vi "Async Initialize.vi"(8 "error in (no error)":errorcluster, 10 "RT Configuration":T1={"Name"="", "Priority"=0, "CAN Session"="", "Frame Count"=0, "Frames"=[], "FPGA Session"=0, "XNET Settings"={"Database"="", "Cluster"="", "Port"="", "Baud rate [Bd]"=0, "Termination"=0, "CAN I/O Mode"=0, "FD Baud rate [Bd]"=500000, "Priority"=100, "Use Legacy"=FALSE, "FD ISO Mode"=0}, "Incoming Frame Session"="", "Incoming Session Invalid"=FALSE, "Incoming Signal Info"={"Signal_Valid_Values"=[], "Signal Names"=[], "Signal Settings Out"=[], "Frame Receive Time Values"=[], "ProtCtr Sig Values"=[]}, "Signal Values"=[]} {"Incoming Signal Info"."Signal Settings Out"."Protection Configuration"."CRC Channels"."Data Type" items=["Signed", "Unsigned", "IEEE Float"]; "XNET Settings"."FD ISO Mode" items=["ISO", "Non ISO", "ISO Legacy"]; "XNET Settings"."CAN I/O Mode" items=["CAN 2.0", "CAN FD", "CAN FD+BRS"]; "XNET Settings"."Termination" items=["Off", "On"]; "Frames"."Protection Configurations"."CRC Channels"."Data Type" items=["Signed", "Unsigned", "IEEE Float"]}, 11 "Process in":refnum<class "Process.lvclass">) -> (0 "error out":errorcluster, 2 "Execute":bool, 3 "Variables":T12={"Process Ref"=refnum, "Comm Ref"=refnum, "Data Refs"={"ProtectionsAndCounters.Ref"=refnum, "Signals.Ref"=refnum, "Status.Ref"=refnum, "Overrides"=refnum, "IncomingSignals.Ref"=refnum, "CtrandProtctnVld.Ref"=refnum, "RcvTime.Ref"=refnum, "TimeDiff.Ref"=refnum, "IncomingProtCtr.Ref"=refnum}, "Settings"={"Name"="", "Priority"=0, "CAN Session"="", "Frame Count"=0, "Frames"=[], "FPGA Session"=0, "XNET Settings"={"Database"="", "Cluster"="", "Port"="", "Baud rate [Bd]"=0, "Termination"=0, "CAN I/O Mode"=0, "FD Baud rate [Bd]"=500000, "Priority"=100, "Use Legacy"=FALSE, "FD ISO Mode"=0}, "Incoming Frame Session"="", "Incoming Session Invalid"=FALSE, "Incoming Signal Info"={"Signal_Valid_Values"=[], "Signal Names"=[], "Signal Settings Out"=[], "Frame Receive Time Values"=[], "ProtCtr Sig Values"=[]}, "Signal Values"=[]}, "Stream Refs"={"Addon"="", "Port"="", "Filter Ref"=refnum, "Default Filter"={"ID Filters"=[], "Direction Filter"=enum."Tx/Rx", "Type Filter"=enum."All"}, "Port Settings"={"Mode"=0, "Baud Rate"=0, "Termination"=0, "FD ISO Mode"=0, "FD Baud Rate"=0}}, "Signal Values"=[], "Incoming Signal Info"={"Signal_Valid_Values"=[], "Signal Names"=[], "Signal Settings Out"=[], "Frame Receive Time Values"=[], "ProtCtr Sig Values"=[]}, "Incoming Frame Session"="", "Incoming Session Invalid"=FALSE} {"Incoming Signal Info"."Signal Settings Out"."Protection Configuration"."CRC Channels"."Data Type" items=["Signed", "Unsigned", "IEEE Float"]; "Stream Refs"."Port Settings"."FD ISO Mode" items=["ISO", "Non ISO", "ISO Legacy"]; "Stream Refs"."Port Settings"."Termination" items=["Off", "On"]; "Stream Refs"."Port Settings"."Mode" items=["CAN 2.0", "CAN FD", "CAN FD+BRS"]; "Settings"."XNET Settings"."FD ISO Mode" items=["ISO", "Non ISO", "ISO Legacy"]; "Settings"."XNET Settings"."CAN I/O Mode" items=["CAN 2.0", "CAN FD", "CAN FD+BRS"]; "Settings"."XNET Settings"."Termination" items=["Off", "On"]})   [LabVIEW 2019, in "Protection and Counter Addon Engine.lvlib"]
uses:
  Protection and Counter Addon Engine.lvlib
  Types/RT Async Engine Variables.ctl
  <vilib>/NI/NIVS Inline Async API/_VS Inline Async API/Process/Process.lvclass
  <vilib>/NI/NI VeriStand Addon Network Comm/Engine/VeriStand Comm.lvclass
  Types/RT Data References.ctl
  <vilib>/NI/NIVS Inline Async API/_Data Access Engine/Data Access Engine/Types/Write.DVR.ctl
  <vilib>/NI/NIVS Inline Async API/_Data Access Engine/Access Type Classes/Write/Write.lvclass
  <vilib>/NI/NIVS Inline Async API/_Data Access Engine/Data Access Engine/Types/Read.DVR.ctl
  <vilib>/NI/NIVS Inline Async API/_Data Access Engine/Access Type Classes/Read/Read.lvclass
  Types/RT Async Engine Settings.ctl
  SubModules/Frame-Protection-Support/Source/Engine/Types/RT Frame Settings.ctl
  SubModules/Frame-Protection-Support/Source/Shared/Types/Exported Frame Type.ctl
  SubModules/Frame-Protection-Support/Source/Engine/Types/RT Protection Configuration.ctl
  SubModules/Frame-Protection-Support/Source/Shared/Types/Protection Type.ctl
  SubModules/Frame-Protection-Support/Source/Shared/Types/XNET Signal Configuration.ctl
  SubModules/Frame-Protection-Support/Source/Shared/Types/Exported Counter Settings.ctl
  SubModules/Frame-Protection-Support/Source/Shared/Types/Exported Event Trigger Type.ctl
  Addon Shared/Types/XNET Settings.ctl
  SubModules/Frame-Protection-Support/Source/Shared/Types/RT_Incoming_Signal_Info.ctl
  SubModules/Frame-Protection-Support/Source/Shared/Types/RT Exported Signal Settings.ctl
  SubModules/CAN-Streaming-Support/Source/Addon/Addon Engine/Types/Engine Stream Refs.ctl
  SubModules/CAN-Streaming-Support/Source/Addon/Addon Shared/Types/Direction Filter.ctl
  SubModules/CAN-Streaming-Support/Source/Addon/Addon Shared/Types/Type Filter.ctl
  SubModules/CAN-Streaming-Support/Source/Addon/Addon Shared/Types/Filter Parameters.ctl
  SubModules/CAN-Streaming-Support/Source/Addon/Addon Engine/Types/Engine Stream Port Settings.ctl
  <vilib>/NI/NI VeriStand Addon Network Comm/Engine/VeriStand Comm.lvclass/VeriStand Comm.ctl
  <vilib>/NI/NIVS Inline Async API/_VS Inline Async API/Process/Process.lvclass/Process.ctl
  <vilib>/NI/NIVS Inline Async API/_VS Inline Async API/Process/Data Member Access/Read Data Access.vi
  <vilib>/NI/NIVS Inline Async API/_VS Inline Async API/Error Handling Process/SubVIs/Error.ConvertArray.vi
  Addon Shared/SubVIs/GUID Lookup.vi
  <vilib>/Utility/SystemLogging/Write to System Log.vi
  <vilib>/NI/AMC/Create Message Queue.vi
  <vilib>/NI/STM/Connection Manager/TCP/Advanced/TCP Initialize Connection Manager (By Reference).vi
  <vilib>/NI/NIVS Inline Async API/_Data Access Engine/Data Access Engine/Methods/Read.Lookup.vi
  <vilib>/NI/NIVS Inline Async API/_Data Access Engine/Data Access Engine/Methods/Write.Lookup.vi
  <vilib>/NI/NIVS Inline Async API/_Data Access Engine/Data Access Engine/Data Access Engine.lvclass
  Addon Shared/Protection and Counter Addon Shared.lvlib
  SubModules/Frame-Protection-Support/Source/Shared/Protection and Counter Support Shared.lvlib
  SubModules/Frame-Protection-Support/Source/Engine/Protection and Counter Support Engine.lvlib
  SubModules/CAN-Streaming-Support/Source/Addon/Addon Shared/CAN Stream Support Shared.lvlib
  SubModules/CAN-Streaming-Support/Source/Addon/Addon Engine/CAN Stream Support Engine.lvlib
  <resource>/objmgr/xnet.rc
  <vilib>/NI VeriStand/Custom Device Tools/Custom Device Utility Library/Custom Device Utility Library.lvlib
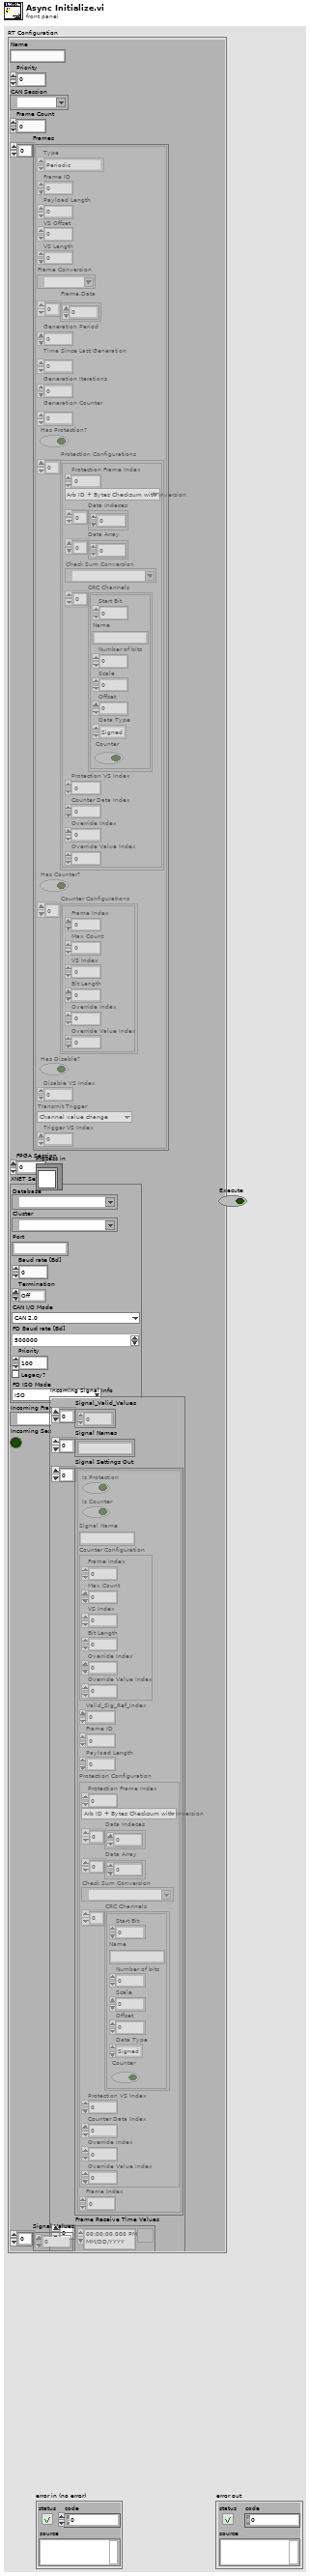
[diagram p1: front panel]
types:
  T1 = typedef "Protection and Counter Addon Engine.lvlib/RT Async Engine Settings.ctl" = cluster{"Name":string, "Priority":i32, "CAN Session":refnum<k21>, "Frame Count":i32, "Frames":T2[], "FPGA Session":u32, "XNET Settings":T9, "Incoming Frame Session":refnum<k21>, "Incoming Session Invalid":bool, "Incoming Signal Info":T10, "Signal Values":dbl[]}
  T2 = typedef "Protection and Counter Support Engine.lvlib/RT Frame Settings.ctl" = cluster{"Type":T3, "Frame ID":u32, "Payload Length":u32, "VS Offset":i32, "VS Length":i32, "Frame Conversion":refnum<k21>, "Frame.Data":dbl[], "Generation Period":u32, "Time Since Last Generation":u32, "Generation Iterations":u32, "Generation Counter":u32, "Has Protection?":bool, "Protection Configurations":T4[], "Has Counter?":bool, "Counter Configurations":T7[], "Has Disable?":bool, "Disable VS Index":i32, "Transmit Trigger":T8, "Trigger VS Index":i32}
  T3 = typedef "Protection and Counter Support Shared.lvlib/Exported Frame Type.ctl" = enum16{"Periodic", "Event", "Periodic/Event"}
  T4 = typedef "Protection and Counter Support Engine.lvlib/RT Protection Configuration.ctl" = cluster{"Protection Frame Index":i32, "Protection Type":T5, "Data Indeces":i32[], "Data Array":dbl[], "Check Sum Conversion":refnum<k21>, "CRC Channels":T6[], "Protection VS Index":i32, "Counter Data Index":i32, "Override Index":i32, "Override Value Index":i32}
  T5 = typedef "Protection and Counter Support Shared.lvlib/Protection Type.ctl" = enum16{"Arb ID + Bytes Checksum with Inversion", "Arb ID + Bytes CRC with Inversion", "Reversed Raw Signal Checksum with Inversion", "Concatenated Two's Compliment"}
  T6 = typedef "Protection and Counter Support Shared.lvlib/XNET Signal Configuration.ctl" = cluster{"Start Bit":i32, "Name":string, "Number of bits":i32, "Scale":dbl, "Offset":dbl, "Data Type":u32, "Counter":bool}
  T7 = typedef "Protection and Counter Support Shared.lvlib/Exported Counter Settings.ctl" = cluster{"Frame Index":i32, "Max Count":dbl, "VS Index":i32, "Bit Length":i64, "Override Index":i32, "Override Value Index":i32}
  T8 = typedef "Protection and Counter Support Shared.lvlib/Exported Event Trigger Type.ctl" = enum16{"Channel value change", "Trigger channel (not zero)", "Channel value change or trigger channel (not zero)", "Trigger channel (any value change)", "Channel value change or trigger channel (any value change)"}
  T9 = typedef "Protection and Counter Addon Shared.lvlib/XNET Settings.ctl" = cluster{"Database":refnum<k21>, "Cluster":refnum<k21>, "Port":string, "Baud rate [Bd]":u64, "Termination":u32, "CAN I/O Mode":u32, "FD Baud rate [Bd]":u64, "Priority":i32, "Use Legacy":bool, "FD ISO Mode":u32}
  T10 = typedef "RT_Incoming_Signal_Info.ctl" = cluster{"Signal_Valid_Values":dbl[], "Signal Names":string[], "Signal Settings Out":T11[], "Frame Receive Time Values":timestamp[], "ProtCtr Sig Values":dbl[]}
  T11 = typedef "RT Exported Signal Settings.ctl" = cluster{"Is Protection":bool, "Is Counter":bool, "Signal Name":string, "Counter Configuration":T7, "Valid_Sig_Ref_Index":i32, "Frame ID":u32, "Payload Length":u32, "Protection Configuration":T4, "Frame Index":i32}
  T12 = typedef "Protection and Counter Addon Engine.lvlib/RT Async Engine Variables.ctl" = cluster{"Process Ref":refnum<class "Process.lvclass">, "Comm Ref":refnum<class "VeriStand Comm.lvclass">, "Data Refs":T13, "Settings":T1, "Stream Refs":T16, "Signal Values":dbl[], "Incoming Signal Info":T10, "Incoming Frame Session":refnum<k21>, "Incoming Session Invalid":bool}
  T13 = typedef "Protection and Counter Addon Engine.lvlib/RT Data References.ctl" = cluster{"ProtectionsAndCounters.Ref":T14, "Signals.Ref":T15, "Status.Ref":T14, "Overrides":T15, "IncomingSignals.Ref":T14, "CtrandProtctnVld.Ref":T14, "RcvTime.Ref":T14, "TimeDiff.Ref":T14, "IncomingProtCtr.Ref":T14}
  T14 = typedef "Data Access Engine.lvlib/Data Access Engine.lvclass/Write.DVR.ctl" = refnum<data-value>
  T15 = typedef "Data Access Engine.lvlib/Data Access Engine.lvclass/Read.DVR.ctl" = refnum<data-value>
  T16 = typedef "CAN Stream Support Engine.lvlib/Engine Stream Refs.ctl" = cluster{"Addon":string, "Port":refnum<k21>, "Filter Ref":refnum<data-value>, "Default Filter":T17, "Port Settings":T20}
  T17 = typedef "CAN Stream Support Shared.lvlib/Filter Parameters.ctl" = cluster{"ID Filters":u32[], "Direction Filter":T18, "Type Filter":T19}
  T18 = typedef "CAN Stream Support Shared.lvlib/Direction Filter.ctl" = enum16{"Tx/Rx", "Rx", "Tx"}
  T19 = typedef "CAN Stream Support Shared.lvlib/Type Filter.ctl" = enum16{"All", "CAN Data", "CAN Remote", "CAN Bus Error", "CAN 2.0 Data", "CAN FD Data", "CAN FD+BRS Data", "J1939 Data", "Delay", "Log Trigger", "Start Trigger"}
  T20 = typedef "CAN Stream Support Engine.lvlib/Engine Stream Port Settings.ctl" = cluster{"Mode":u32, "Baud Rate":u64, "Termination":u32, "FD ISO Mode":u32, "FD Baud Rate":u64}
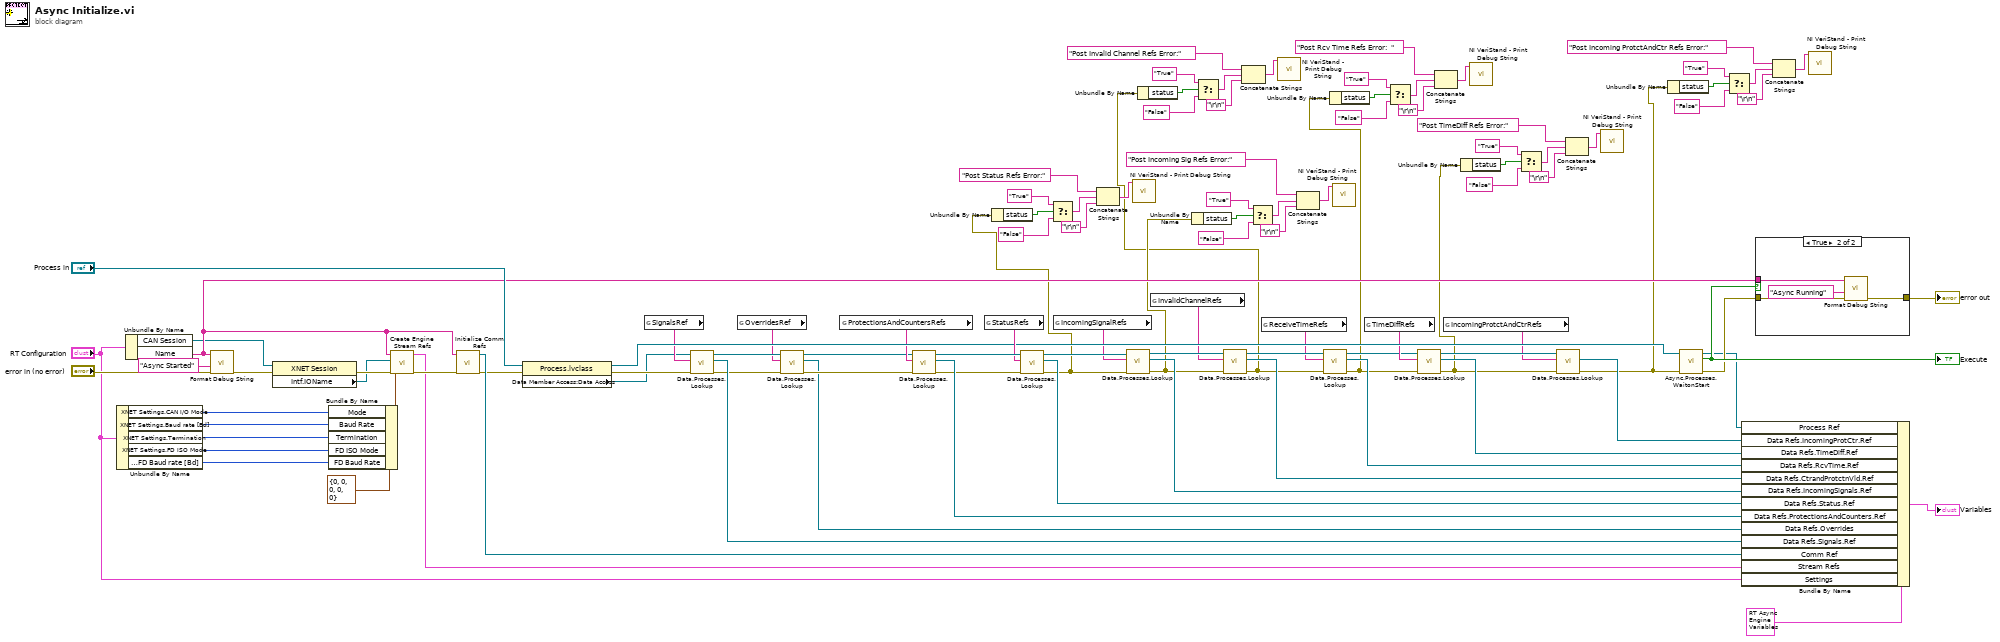
[diagram p0: block diagram]
diagram:
  n1 = Unbundle By Name("RT Configuration") -> ("XNET Settings.CAN I/O Mode"=w69:u32, "XNET Settings.Baud rate [Bd]"=w66:u64, "XNET Settings.Termination"=w67:u32, "XNET Settings.FD ISO Mode"=w65:u32, "XNET Settings.FD Baud rate [Bd]"=w68:u64)
  n2 = Unbundle By Name("RT Configuration") -> ("CAN Session"=w81:refnum<k21>, "Name"=w82:string)
  n3 = call "Format Debug String.vi"("error in (no error)"="error in (no error)", "State"="Async Started", "Name"=w82) -> ("error out"=w84:errorcluster)  [unwired: 8 in]
  n4 = property class="XNET Session"(reference=w81, error in=w84) -> (error out=w83:errorcluster, "Intf.IOName"=w80:refnum<k21>)  [unwired: 1 out]
  n5 = Bundle By Name(cluster=T20 {"Mode"=0, "Baud Rate"=0, "Termination"=0, "FD ISO Mode"=0, "FD Baud Rate"=0} ("Port Settings"), "Mode"=w69, "Baud Rate"=w66, "Termination"=w67, "FD ISO Mode"=w65, "FD Baud Rate"=w68) -> (w70:T20)
  n6 = call "Create Engine Stream Refs.vi"("error in (no error)"=w83, "Port Settings"=w70, "Port"=w80, "Addon"=w82) -> ("error out"=w85:errorcluster, "Refs"=w79:T16)  [unwired: 6 in]
  n7 = call <vilib>:"Initialize Comm Refs.vi"("error in (no error)"=w85, "Name"=w82) -> ("error out"=w100:errorcluster, "Comm.lvclass"=w106:refnum<class "VeriStand Comm.lvclass">)  [unwired: 8 in]
  n8 = property class="Process.lvclass"(reference="Process in", error in=w100) -> (reference out=w91:refnum<class "Process.lvclass">, error out=w88:errorcluster, "Data Member Access:Data Access"=w87:refnum<class "Data Access Engine.lvclass">)
  n9 = global read "GUID Lookup.vi" "SignalsRef"() -> (w89:string)
  n10 = call-poly <vilib>:"Data.Processes.Lookup.vi"("error in (no error)"=w88, "Name"=w89, "Data Access API in"=w87) -> ("error out"=w78:errorcluster, "Ref"=w105:T15, "Data Access API out"=w76:refnum<class "Data Access Engine.lvclass">)  [unwired: 5 in, 1 out]
  n11 = global read "GUID Lookup.vi" "OverridesRef"() -> (w74:string)
  n12 = call-poly <vilib>:"Data.Processes.Lookup.vi"("error in (no error)"=w78, "Name"=w74, "Data Access API in"=w76) -> ("error out"=w77:errorcluster, "Ref"=w73:T15, "Data Access API out"=w75:refnum<class "Data Access Engine.lvclass">)  [unwired: 5 in, 1 out]
  n13 = global read "GUID Lookup.vi" "ProtectionsAndCountersRefs"() -> (w90:string)
  n14 = call-poly <vilib>:"Data.Processes.Lookup.vi"("error in (no error)"=w77, "Name"=w90, "Data Access API in"=w75) -> ("error out"=w94:errorcluster, "Ref"=w104:T14, "Data Access API out"=w93:refnum<class "Data Access Engine.lvclass">)  [unwired: 5 in, 1 out]
  n15 = global read "GUID Lookup.vi" "StatusRefs"() -> (w92:string)
  n16 = call-poly <vilib>:"Data.Processes.Lookup.vi"("error in (no error)"=w94, "Name"=w92, "Data Access API in"=w93) -> ("error out"=w41:errorcluster, "Ref"=w103:T14, "Data Access API out"=w64:refnum<class "Data Access Engine.lvclass">)  [unwired: 5 in, 1 out]
  n17 = Unbundle By Name(w41) -> ("status"=w45:bool)
  n18 = Select(t="True" ("string"), s=w45, f="False" ("string")) -> (s? t:f=w42:string)
  n19 = global read "GUID Lookup.vi" "IncomingSignalRefs"() -> (w61:string)
  n20 = Concatenate Strings("Post Status Refs Error:" ("string"), w42, "\r\n") -> (w47:string)
  n21 = call-poly <vilib>:"Data.Processes.Lookup.vi"("error in (no error)"=w41, "Name"=w61, "Data Access API in"=w64) -> ("error out"=w33:errorcluster, "Ref"=w55:T14, "Data Access API out"=w63:refnum<class "Data Access Engine.lvclass">)  [unwired: 5 in, 1 out]
  n22 = call <vilib>:"NI VeriStand - Print Debug String.vi"("Message"=w47) -> ()  [unwired: 10 in, 1 out]
  n23 = global read "GUID Lookup.vi" "InvalidChannelRefs"() -> (w60:string)
  n24 = Unbundle By Name(w33) -> ("status"=w37:bool)
  n25 = call-poly <vilib>:"Data.Processes.Lookup.vi"("error in (no error)"=w33, "Name"=w60, "Data Access API in"=w63) -> ("error out"=w4:errorcluster, "Ref"=w57:T14, "Data Access API out"=w62:refnum<class "Data Access Engine.lvclass">)  [unwired: 5 in, 1 out]
  n26 = Unbundle By Name(w4) -> ("status"=w29:bool)
  n27 = Select(t="True" ("string"), s=w29, f="False" ("string")) -> (s? t:f=w26:string)
  n28 = Concatenate Strings("Post Invalid Channel Refs Error:" ("string"), w26, "\r\n") -> (w31:string)
  n29 = Select(t="True" ("string"), s=w37, f="False" ("string")) -> (s? t:f=w34:string)
  n30 = global read "GUID Lookup.vi" "ReceiveTimeRefs"() -> (w59:string)
  n31 = call <vilib>:"NI VeriStand - Print Debug String.vi"("Message"=w31) -> ()  [unwired: 10 in, 1 out]
  n32 = Concatenate Strings("Post Incoming Sig Refs Error:" ("string"), w34, "\r\n") -> (w39:string)
  n33 = call-poly <vilib>:"Data.Processes.Lookup.vi"("error in (no error)"=w4, "Name"=w59, "Data Access API in"=w62) -> ("error out"=w3:errorcluster, "Ref"=w56:T14, "Data Access API out"=w53:refnum<class "Data Access Engine.lvclass">)  [unwired: 5 in, 1 out]
  n34 = Unbundle By Name(w3) -> ("status"=w22:bool)
  n35 = call <vilib>:"NI VeriStand - Print Debug String.vi"("Message"=w39) -> ()  [unwired: 10 in, 1 out]
  n36 = global read "GUID Lookup.vi" "TimeDiffRefs"() -> (w54:string)
  n37 = Select(t="True" ("string"), s=w22, f="False" ("string")) -> (s? t:f=w19:string)
  n38 = call-poly <vilib>:"Data.Processes.Lookup.vi"("error in (no error)"=w3, "Name"=w54, "Data Access API in"=w53) -> ("error out"=w2:errorcluster, "Ref"=w52:T14, "Data Access API out"=w51:refnum<class "Data Access Engine.lvclass">)  [unwired: 5 in, 1 out]
  n39 = Concatenate Strings("Post Rcv Time Refs Error:  " ("string"), w19, "\r\n") -> (w24:string)
  n40 = global read "GUID Lookup.vi" "IncomingProtctAndCtrRefs"() -> (w50:string)
  n41 = Unbundle By Name(w2) -> ("status"=w15:bool)
  n42 = call <vilib>:"NI VeriStand - Print Debug String.vi"("Message"=w24) -> ()  [unwired: 10 in, 1 out]
  n43 = Select(t="True" ("string"), s=w15, f="False" ("string")) -> (s? t:f=w12:string)
  n44 = call-poly <vilib>:"Data.Processes.Lookup.vi"("error in (no error)"=w2, "Name"=w50, "Data Access API in"=w51) -> ("error out"=w1:errorcluster, "Ref"=w49:T14)  [unwired: 5 in, 2 out]
  n45 = Concatenate Strings("Post TimeDiff Refs Error:" ("string"), w12, "\r\n") -> (w17:string)
  n46 = call <vilib>:"NI VeriStand - Print Debug String.vi"("Message"=w17) -> ()  [unwired: 10 in, 1 out]
  n47 = Unbundle By Name(w1) -> ("status"=w8:bool)
  n48 = call <vilib>:"Async.Processes.WaitonStart.vi"("error in (no error)"=w1, "Process"=w91) -> ("error out"=w97:errorcluster, "Execute"=w99:bool, "Process out"=w58:refnum<class "Process.lvclass">)  [unwired: 7 in]
  "Execute" <- w99
  n49 = Select(t="True" ("string"), s=w8, f="False" ("string")) -> (s? t:f=w5:string)
  n50 = Bundle By Name(cluster=T12 {"Process Ref"=refnum, "Comm Ref"=refnum, "Data Refs"={"ProtectionsAndCounters.Ref"=refnum, "Signals.Ref"=refnum, "Status.Ref"=refnum, "Overrides"=refnum, "IncomingSignals.Ref"=refnum, "CtrandProtctnVld.Ref"=refnum, "RcvTime.Ref"=refnum, "TimeDiff.Ref"=refnum, "IncomingProtCtr.Ref"=refnum}, "Settings"={"Name"="", "Priority"=0, "CAN Session"="", "Frame Count"=0, "Frames"=[], "FPGA Session"=0, "XNET Settings"={"Database"="", "Cluster"="", "Port"="", "Baud rate [Bd]"=0, "Termination"=0, "CAN I/O Mode"=0, "FD Baud rate [Bd]"=500000, "Priority"=100, "Use Legacy"=FALSE, "FD ISO Mode"=0}, "Incoming Frame Session"="", "Incoming Session Invalid"=FALSE, "Incoming Signal Info"={"Signal_Valid_Values"=[], "Signal Names"=[], "Signal Settings Out"=[], "Frame Receive Time Values"=[], "ProtCtr Sig Values"=[]}, "Signal Values"=[]}, "Stream Refs"={"Addon"="", "Port"="", "Filter Ref"=refnum, "Default Filter"={"ID Filters"=[], "Direction Filter"=enum."Tx/Rx", "Type Filter"=enum."All"}, "Port Settings"={"Mode"=0, "Baud Rate"=0, "Termination"=0, "FD ISO Mode"=0, "FD Baud Rate"=0}}, "Signal Values"=[], "Incoming Signal Info"={"Signal_Valid_Values"=[], "Signal Names"=[], "Signal Settings Out"=[], "Frame Receive Time Values"=[], "ProtCtr Sig Values"=[]}, "Incoming Frame Session"="", "Incoming Session Invalid"=FALSE}, "Process Ref"=w58, "Data Refs.IncomingProtCtr.Ref"=w49, "Data Refs.TimeDiff.Ref"=w52, "Data Refs.RcvTime.Ref"=w56, "Data Refs.CtrandProtctnVld.Ref"=w57, "Data Refs.IncomingSignals.Ref"=w55, "Data Refs.Status.Ref"=w103, "Data Refs.ProtectionsAndCounters.Ref"=w104, "Data Refs.Overrides"=w73, "Data Refs.Signals.Ref"=w105, "Comm Ref"=w106, "Stream Refs"=w79, "Settings"="RT Configuration") -> (→"Variables":T12)
  n51 = case shown="True" w99 {
    tunnel: w97 -> [w107 w110]
    tunnel: [w107 w109] -> w98
    tunnel: w82 -> [_ w108]
    frame False {
    }
    frame True {
      n52 = call "Format Debug String.vi"("error in (no error)"=w110, "State"="Async Running", "Name"=w108) -> ("error out"=w109:errorcluster)  [unwired: 8 in]
    }
  }
  "error out" <- w98
  n53 = Concatenate Strings("Post Incoming ProtctAndCtr Refs Error:" ("string"), w5, "\r\n") -> (w10:string)
  n54 = call <vilib>:"NI VeriStand - Print Debug String.vi"("Message"=w10) -> ()  [unwired: 10 in, 1 out]
